vi "execute.vi"(8 "error in (no error)":errorcluster, 10 "Context in":refnum<class "Context.lvclass">, 11 "ClearAOSCorrectionCommand in":refnum<class "ClearAOSCorrectionCommand.lvclass">) -> (0 "error out":errorcluster, 2 "Context out":refnum<class "Context.lvclass">, 3 "ClearAOSCorrectionCommand out":refnum<class "ClearAOSCorrectionCommand.lvclass">)   [LabVIEW 2016, in "ClearAOSCorrectionCommand.lvclass"]
uses:
  ClearAOSCorrectionCommand.lvclass
  Context/Context.lvclass
  ClearAOSCorrectionCommand.lvclass/ClearAOSCorrectionCommand.ctl
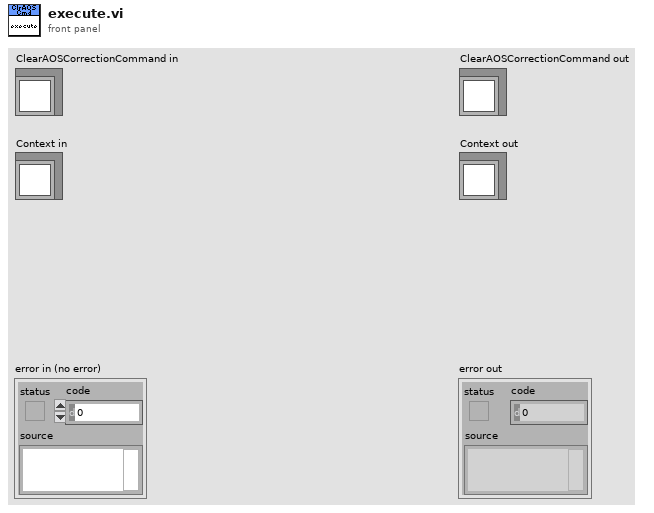
[diagram p1: front panel]
types:
  T1 = typedef "M1M3SupportTopics.lvlib/CommandClearAOSCorrection.ctl" = cluster{"CommandId":T2, "ClearAOSCorrection":bool}
  T2 = typedef "M1M3SupportTopics.lvlib/CommandId.ctl" = i32
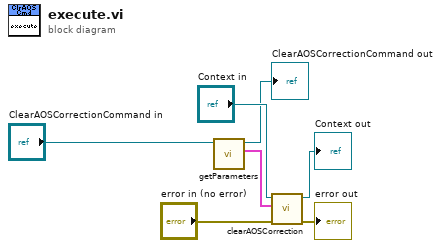
[diagram p0: block diagram]
diagram:
  n1 = call "getParameters.vi"("ClearAOSCorrectionCommand in"="ClearAOSCorrectionCommand in") -> ("Parameters"=w5:T1, "ClearAOSCorrectionCommand out"=→"ClearAOSCorrectionCommand out":refnum<class "ClearAOSCorrectionCommand.lvclass">)  [unwired: 9 in]
  n2 = call-dynamic "clearAOSCorrection.vi"("error in (no error)"="error in (no error)", "Parameters"=w5, "Context in"="Context in") -> ("error out"=→"error out":errorcluster, "Context out"=→"Context out":refnum<class "Context.lvclass">)  [unwired: 7 in]
